vi "Controller_Thread.vi"(9 "user event":refnum<user-event>, 10 "controller queue in":refnum<queue>, 11 "ble queue out":refnum<queue>) -> ()   [LabVIEW 2020]
uses:
  BLE_Request.ctl
  BLE_Request_Command.ctl
  Controller_Request.ctl
  Controller_Request_Command.ctl
  Controller_Response.ctl
  Controller_Response_Command.ctl
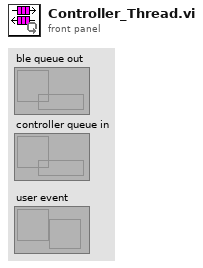
[diagram p1: front panel]
types:
  T1 = typedef "Controller_Request.ctl" = cluster{"Command":T2, "Parameter":variant}
  T2 = typedef "Controller_Request_Command.ctl" = enum16{"BLE_ScannedDevices", "BLE_ConnectionResult", "BLE_NotificationToogleResult", "BLE_NotificationData", "BLE_ConnTimeout", "BLE_CloseResult", "User_Init", "User_ScanRequest", "User_ConnectionRequest", "User_CloseRequest", "User_NotficationToggleRequest"}
  T3 = typedef "Controller_Response.ctl" = cluster{"Command":T4, "Parameter":variant}
  T4 = typedef "Controller_Response_Command.ctl" = enum16{"Init", "ScanResult", "ConnectionResult", "ConnectionTimeout", "NotificationToogleResult", "NotificationData", "CloseResult"}
  T5 = typedef "BLE_Request.ctl" = cluster{"Command":T6, "Parameter":variant}
  T6 = typedef "BLE_Request_Command.ctl" = enum16{"BLE_Idle", "BLE_Init", "BLE_ScanToogle", "BLE_Connect", "BLE_NotificationToogle", "BLE_Close"}
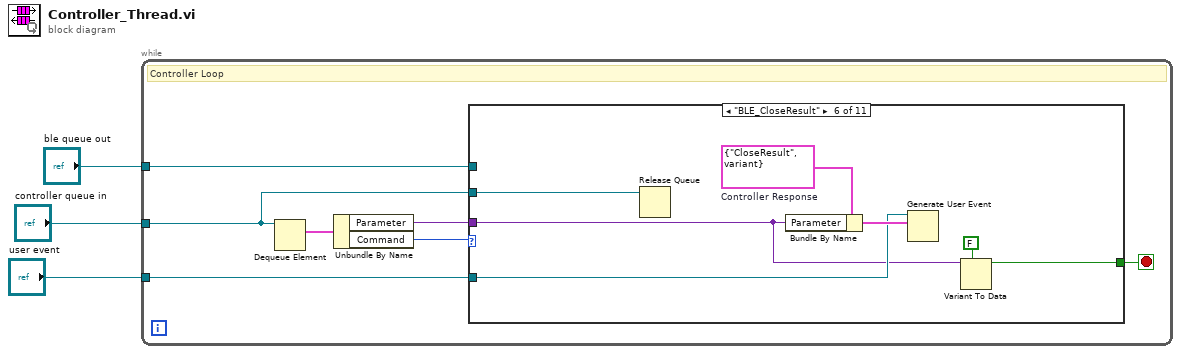
[diagram p0: block diagram]
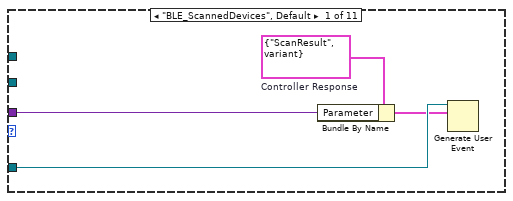
[diagram p2: hidden frame]
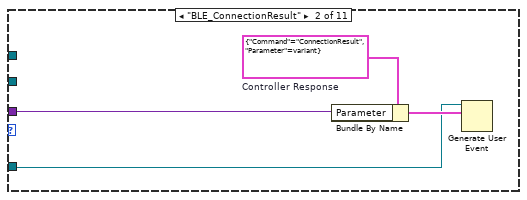
[diagram p3: hidden frame]
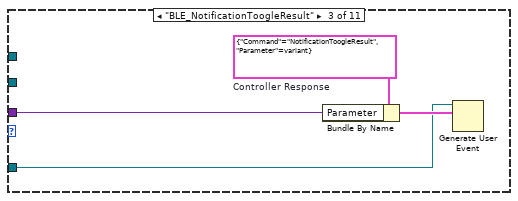
[diagram p4: hidden frame]
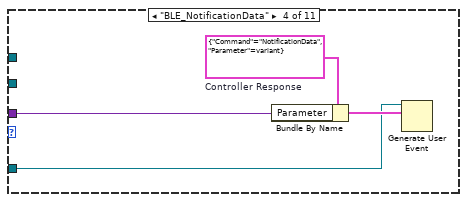
[diagram p5: hidden frame]
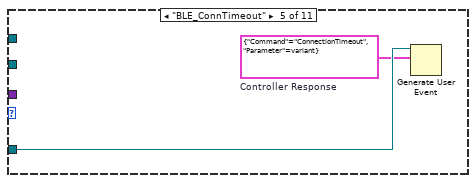
[diagram p6: hidden frame]
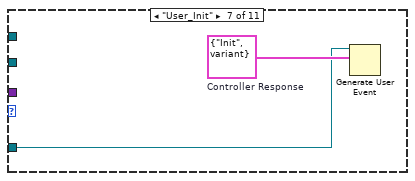
[diagram p7: hidden frame]
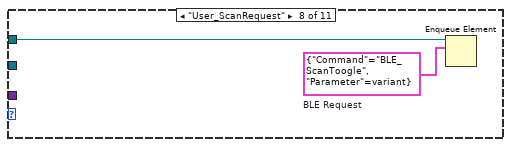
[diagram p8: hidden frame]
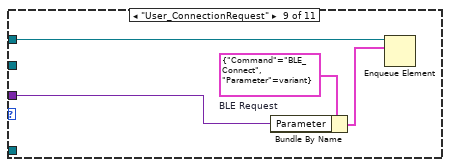
[diagram p9: hidden frame]
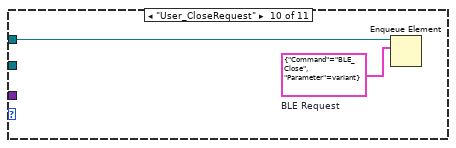
[diagram p10: hidden frame]
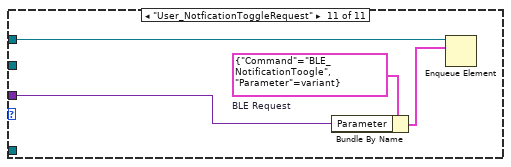
[diagram p11: hidden frame]
diagram:
  n1 = while {
    tunnel: "ble queue out" -> [w7]
    tunnel: "controller queue in" -> [w4]
    tunnel: "user event" -> [w6]
    stop <- w5 stop-if-true
    # "Controller Loop"
    n2 = Dequeue Element(queue=w4) -> (element=w10:T1)  [unwired: 2 in, 3 out]
    n3 = Unbundle By Name(w10) -> ("Parameter"=w8:variant, "Command"=w9:T2)
    n4 = case shown="\"BLE_CloseResult\"" w9 {
      tunnel: w8 -> [w11 w15 w19 w24 _ w32 _ _ w40 _ w46]
      tunnel: w7 -> [_ _ _ _ _ _ _ w39 w43 w44 w47]
      tunnel: w6 -> [w14 w16 w20 w23 w28 w33 w36 _ _ _ _]
      tunnel: [_ _ _ _ _ w30 _ _ _ _ _] -> w5
      tunnel: w4 -> [_ _ _ _ _ w29 _ _ _ _ _]
      frame "BLE_ScannedDevices", Default {
        w12 = T3 {"Command"=enum."ScanResult", "Parameter"=variant}  # Controller Response
        n5 = Bundle By Name(cluster=w12, "Parameter"=w11) -> (w13:T3)
        n6 = Generate User Event(user event=w14, event data cluster=w13) -> ()  [unwired: 2 in, 2 out]
      }
      frame "BLE_ConnectionResult" {
        w17 = T3 {"Command"=enum."ConnectionResult", "Parameter"=variant}  # Controller Response
        n7 = Bundle By Name(cluster=w17, "Parameter"=w15) -> (w18:T3)
        n8 = Generate User Event(user event=w16, event data cluster=w18) -> ()  [unwired: 2 in, 2 out]
      }
      frame "BLE_NotificationToogleResult" {
        w21 = T3 {"Command"=enum."NotificationToogleResult", "Parameter"=variant}  # Controller Response
        n9 = Bundle By Name(cluster=w21, "Parameter"=w19) -> (w22:T3)
        n10 = Generate User Event(user event=w20, event data cluster=w22) -> ()  [unwired: 2 in, 2 out]
      }
      frame "BLE_NotificationData" {
        w25 = T3 {"Command"=enum."NotificationData", "Parameter"=variant}  # Controller Response
        n11 = Bundle By Name(cluster=w25, "Parameter"=w24) -> (w26:T3)
        n12 = Generate User Event(user event=w23, event data cluster=w26) -> ()  [unwired: 2 in, 2 out]
      }
      frame "BLE_ConnTimeout" {
        w27 = T3 {"Command"=enum."ConnectionTimeout", "Parameter"=variant}  # Controller Response
        n13 = Generate User Event(user event=w28, event data cluster=w27) -> ()  [unwired: 2 in, 2 out]
      }
      frame "BLE_CloseResult" {
        w34 = T3 {"Command"=enum."CloseResult", "Parameter"=variant}  # Controller Response
        n14 = Release Queue(queue=w29) -> ()  [unwired: 2 in, 3 out]
        n15 = Bundle By Name(cluster=w34, "Parameter"=w32) -> (w35:T3)
        n16 = Generate User Event(user event=w33, event data cluster=w35) -> ()  [unwired: 2 in, 2 out]
        n17 = Variant To Data(type=FALSE, Variant=w32) -> (data=w30:bool)  [unwired: 1 in, 1 out]
      }
      frame "User_Init" {
        w37 = T3 {"Command"=enum."Init", "Parameter"=variant}  # Controller Response
        n18 = Generate User Event(user event=w36, event data cluster=w37) -> ()  [unwired: 2 in, 2 out]
      }
      frame "User_ScanRequest" {
        w38 = T5 {"Command"=enum."BLE_ScanToogle", "Parameter"=variant}  # BLE Request
        n19 = Enqueue Element(queue=w39, element=w38) -> ()  [unwired: 2 in, 3 out]
      }
      frame "User_ConnectionRequest" {
        w42 = T5 {"Command"=enum."BLE_Connect", "Parameter"=variant}  # BLE Request
        n20 = Bundle By Name(cluster=w42, "Parameter"=w40) -> (w41:T5)
        n21 = Enqueue Element(queue=w43, element=w41) -> ()  [unwired: 2 in, 3 out]
      }
      frame "User_CloseRequest" {
        w45 = T5 {"Command"=enum."BLE_Close", "Parameter"=variant}  # BLE Request
        n22 = Enqueue Element(queue=w44, element=w45) -> ()  [unwired: 2 in, 3 out]
      }
      frame "User_NotficationToggleRequest" {
        w48 = T5 {"Command"=enum."BLE_NotificationToogle", "Parameter"=variant}  # BLE Request
        n23 = Bundle By Name(cluster=w48, "Parameter"=w46) -> (w49:T5)
        n24 = Enqueue Element(queue=w47, element=w49) -> ()  [unwired: 2 in, 3 out]
      }
    }
  }
